vi "LockinDAQ.Stop.vi"(8 "error in (no error)":errorcluster, 11 "LockinDAQ":refnum<class "LockinDAQ.lvclass">) -> (0 "error out":errorcluster, 3 "LockinDAQ out":refnum<class "LockinDAQ.lvclass">)   [LabVIEW 2016, in "LockinDAQ.lvclass"]
uses:
  LockinDAQ.lvclass
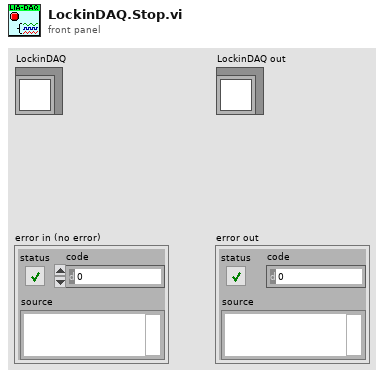
[diagram p1: front panel]
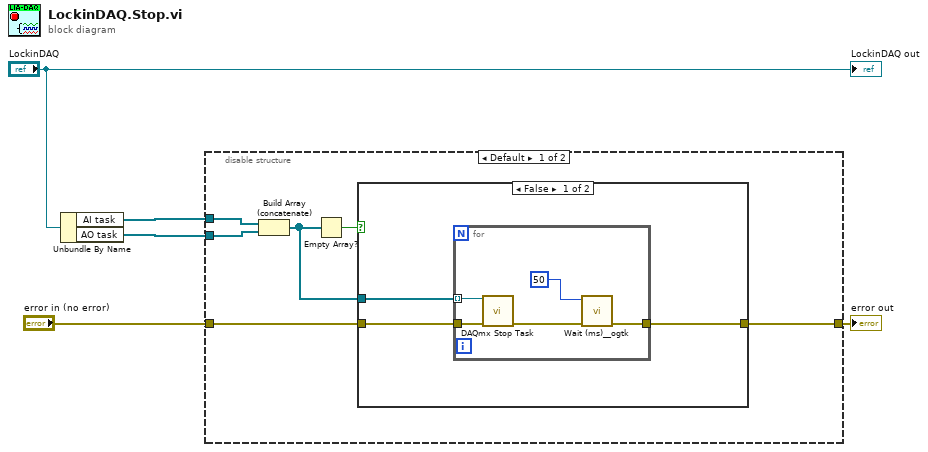
[diagram p0: block diagram]
diagram:
  n1 = Unbundle By Name("LockinDAQ") -> ("AI task"=w2:refnum<k21>[], "AO task"=w3:refnum<k21>[])
  n2 = disable-structure shown="Default" {
    disable-tunnel: "error in (no error)" -> [w11 _]
    disable-tunnel: [w8 _] -> w4
    disable-tunnel: w3 -> [w9 _]
    disable-tunnel: w2 -> [w10 _]
    frame condition #0 (active) {
      n3 = Build Array (concatenate)(w10, w9) -> (w6:refnum<k21>[])
      n4 = Empty Array?(array=w6) -> (empty?=w7:bool)
      n5 = case shown="False" w7 {
        tunnel: w11 -> [w14 w20]
        tunnel: w6 -> [w13 _]
        tunnel: [w12 w20] -> w8
        frame False {
          n6 = for {
            tunnel: w13 -> [w19] mode=indexing
            tunnel: w14 -> [w18]
            tunnel: [w16] -> w12
            n7 = call <vilib>:"DAQmx Stop Task.vi"("task/channels in"=w19, "error in"=w18) -> ("error out"=w17:errorcluster)  [unwired: 12 in, 1 out]
            n8 = call <userlib>:"Wait (ms)__ogtk.vi"("error in (no error)"=w17, "milliseconds to wait"=u32 50) -> ("error out"=w16:errorcluster)  [unwired: 8 in, 1 out]
          }
        }
        frame True {
        }
      }
    }
    frame condition #1 {
    }
  }
  "error out" <- w4
  "LockinDAQ out" <- "LockinDAQ"
